vi "Date Trigger.vi"(11 "y":u32) -> ()   [LabVIEW 2018]
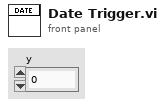
[diagram p1: front panel]
types:
  T1 = typedef "LVDateTimeRec.ctl" = cluster{"fractional second":dbl, "second":i32, "minute":i32, "hour":i32, "day of month":i32, "month":i32, "year":i32, "day of week":i32, "day of year":i32, "DST":i32}
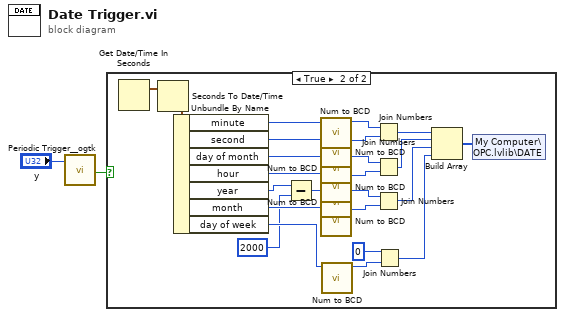
[diagram p0: block diagram]
diagram:
  n1 = call <userlib>:"Periodic Trigger__ogtk.vi"("time (ms)"="y") -> ("Triggered"=w2:bool)  [unwired: 12 in, 2 out]
  n2 = case shown="True" w2 {
    frame False {
    }
    frame True {
      n3 = Get Date/Time In Seconds() -> (seconds since 1Jan1904=w26:timestamp)
      n4 = Seconds To Date/Time(time stamp (now)=w26) -> (date time rec=w25:T1)  [unwired: 1 in]
      n5 = Unbundle By Name(w25) -> ("minute"=w24:i32, "second"=w23:i32, "day of month"=w16:i32, "hour"=w15:i32, "year"=w4:i32, "month"=w14:i32, "day of week"=w12:i32)
      n6 = Subtract(x=w4, y=2000) -> (x-y=w5:i32)
      n7 = call "Num to BCD.vi"("Numeric"=w24) -> ("BCD"=w21:u8)  [unwired: 10 in]
      n8 = call "Num to BCD.vi"("Numeric"=w23) -> ("BCD"=w22:u8)  [unwired: 10 in]
      n9 = call "Num to BCD.vi"("Numeric"=w16) -> ("BCD"=w20:u8)  [unwired: 10 in]
      n10 = call "Num to BCD.vi"("Numeric"=w15) -> ("BCD"=w19:u8)  [unwired: 10 in]
      n11 = call "Num to BCD.vi"("Numeric"=w5) -> ("BCD"=w17:u8)  [unwired: 10 in]
      n12 = call "Num to BCD.vi"("Numeric"=w14) -> ("BCD"=w18:u8)  [unwired: 10 in]
      n13 = call "Num to BCD.vi"("Numeric"=w12) -> ("BCD"=w13:u8)  [unwired: 10 in]
      n14 = Join Numbers(hi=w21, lo=w22) -> ((hi.lo)=w10:u16)
      n15 = Join Numbers(hi=w20, lo=w19) -> ((hi.lo)=w9:u16)
      n16 = Join Numbers(hi=w17, lo=w18) -> ((hi.lo)=w8:u16)
      n17 = Join Numbers(hi=u8 0, lo=w13) -> ((hi.lo)=w7:u16)
      n18 = Build Array(w10, w9, w8, w7) -> (w6:u16[])
      n19 = shared-variable "My Computer\\OPC.lvlib\\DATE"(w6) -> ()  [unwired: 1 in, 1 out]
    }
  }
